vi "Construct.vi"(8 "series":i32(ring)=2 items=["AM", "H3U", "H5U"], 9 "port":i32=502, 10 "station":u8=1, 11 "ipAddress":string="192.168.1.88") -> (3 "MelsecMcNet out":refnum<class "InovanceModbusTcp.lvclass">)   [LabVIEW 2020, in "HslCommunication.lvlib" / "InovanceModbusTcp.lvclass"]
uses:
  InovanceModbusTcp.lvclass
  InovanceModbusTcp.lvclass/InovanceModbusTcp.ctl
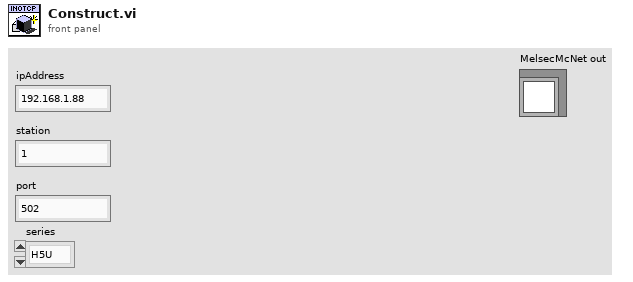
[diagram p1: front panel]
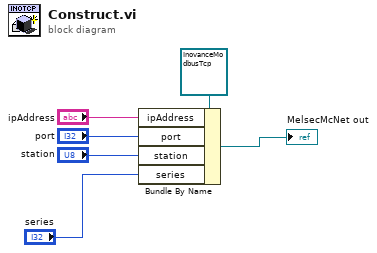
[diagram p0: block diagram]
diagram:
  n1 = Bundle By Name(cluster=refnum<class "InovanceModbusTcp.lvclass"> refnum ("MelsecMcNet in"), "ipAddress"="ipAddress", "port"="port", "station"="station", "series"="series") -> (→"MelsecMcNet out":refnum<class "InovanceModbusTcp.lvclass">)
